vi "GEOM_GetModifiers.vi"(8 "error in (no error)":errorcluster) -> (0 "error out":errorcluster, 2 "GEOM_modifiers":T1={"Binning"={"x"=1, "y"=1}, "sections"=[]} {"Binning"."y" min=1; "Binning"."x" min=1})   [LabVIEW 2016]
uses:
  private/vis/GEOM_AmpModifiers.ctl
  private/vis/GEOM_Binning.ctl
  private/vis/GEOM_Moifier.ctl
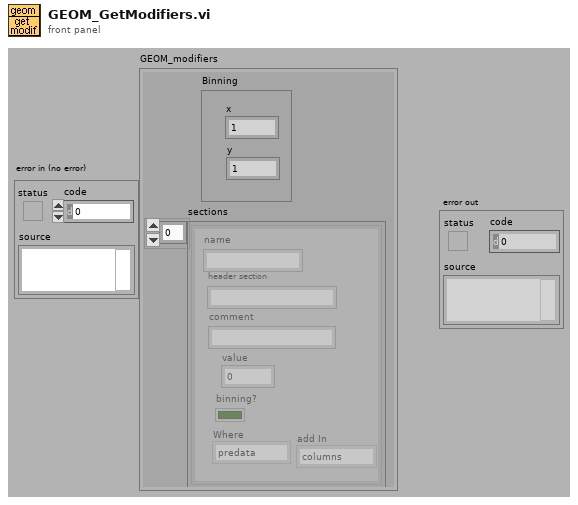
[diagram p1: front panel]
types:
  T1 = typedef "GEOM_AmpModifiers.ctl" = cluster{"Binning":T2, "sections":T3[]}
  T2 = typedef "GEOM_Binning.ctl" = cluster{"x":u32, "y":u32}
  T3 = typedef "GEOM_Moifier.ctl" = cluster{"name":string, "header section":string, "comment":string, "value":i32, "binning?":bool, "Where":enum16{"predata", "postdata"}, "add In":enum16{"columns", "rows", "none"}}
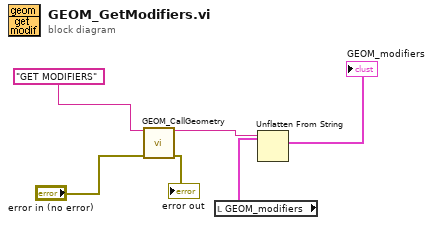
[diagram p0: block diagram]
diagram:
  n1 = call "GEOM_CallGeometry.vi"("Command"="GET MODIFIERS", "error in (no error)"="error in (no error)") -> ("ImmedReplyString"=w6:string, "error out"=→"error out":errorcluster)  [unwired: 12 out]
  n2 = local read "GEOM_modifiers"() -> (w2:T1)
  n3 = Unflatten From String(type=w2, binary string=w6) -> (value=→"GEOM_modifiers":T1)  [unwired: 1 in, 4 out]
